vi "Send Packet.vi"(6 "timeout (0ms : no ack)":i32, 8 "error in (no error)":errorcluster, 10 "Packet":refnum<class "ControlPacket.lvclass">, 11 "Session in":refnum<class "Session.lvclass">) -> (0 "error out":errorcluster, 1 "validated":bool, 2 "Response":refnum<class "ControlPacket.lvclass">[](array[class]), 3 "Session out":refnum<class "Session.lvclass">)   [LabVIEW 2013, in "MQTT Server.lvlib" / "Session.lvclass"]
uses:
  Session.lvclass
  Control Packets/ControlPacket/ControlPacket.lvclass
  MQTT_Base/Response -- cluster.ctl
  Session.lvclass/Session.ctl
  MQTT_Base/MQTT_Base.lvclass
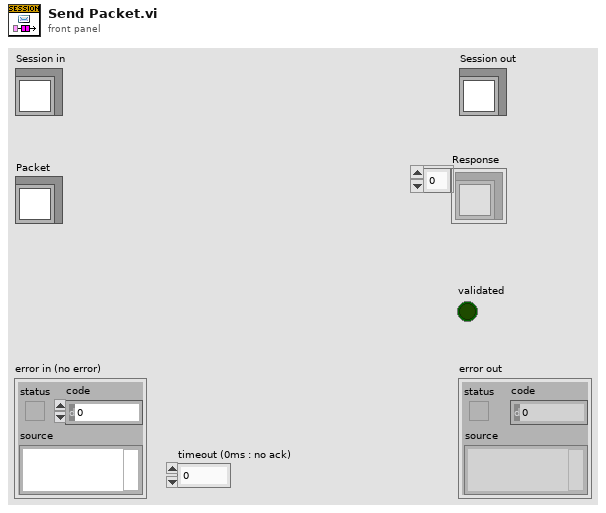
[diagram p1: front panel]
types:
  T1 = typedef "MQTT Server.lvlib/MQTT_Base.lvclass/Response -- cluster.ctl" = cluster{"Packet":refnum<class "ControlPacket.lvclass">, "Protocol Error":errorcluster, "disconnect session":bool, "[ACK]":refnum<notifier>[]}
  T2 = typedef "ControlPacket.lvclass/Control Packet Type -- enum.ctl" = enum16{"Reserved", "CONNECT", "CONNACK", "PUBLISH", "PUBACK", "PUBREC", "PUBREL", "PUBCOMP", "SUBSCRIBE", "SUBACK", "UNSUBSCRIBE", "UNSUBACK", "PINGREQ", "PINGRESP", "DISCONNECT", "Reserved(15)"}
  T3 = typedef "ControlPacket.lvclass/QualityOfService -- enum.ctl" = enum16{"0 (At Most Once)", "1 (At Least Once)", "2 (Exactly Once)"}
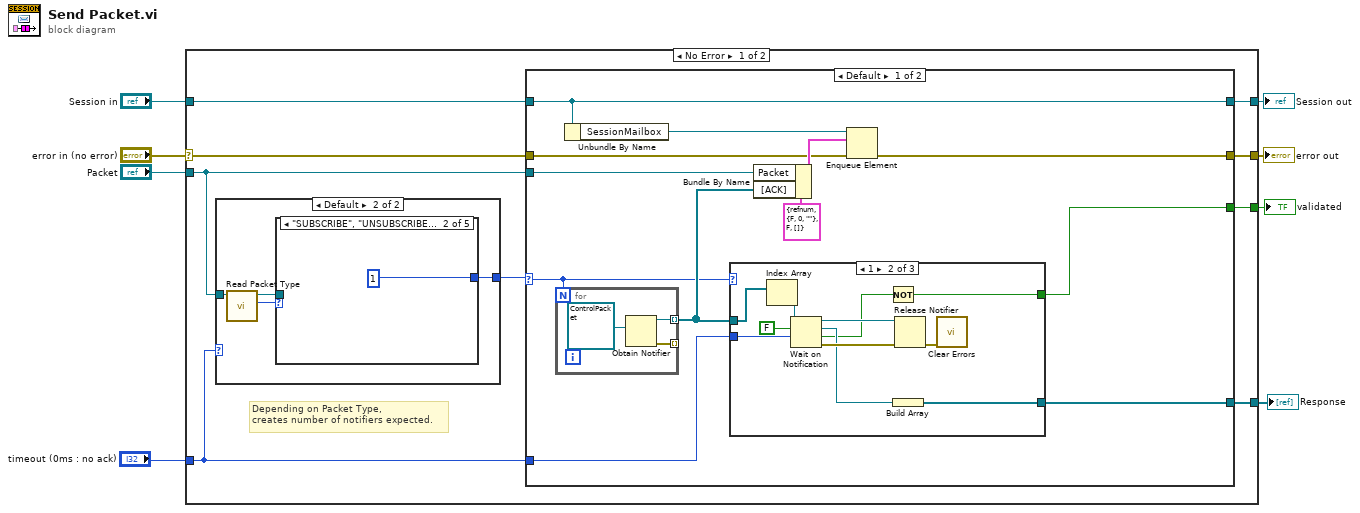
[diagram p0: block diagram]
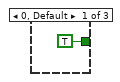
[diagram p2: hidden frame]
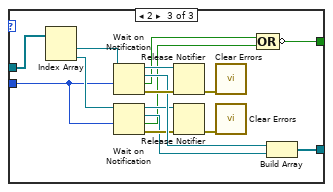
[diagram p3: hidden frame]
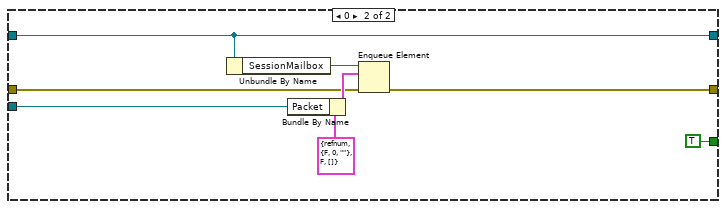
[diagram p4: hidden frame]
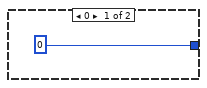
[diagram p5: hidden frame]
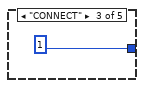
[diagram p7: hidden frame]
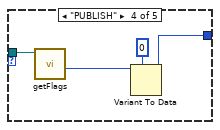
[diagram p8: hidden frame]
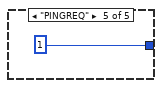
[diagram p9: hidden frame]
diagram:
  n1 = case shown="No Error" "error in (no error)" {
    selector: "error in (no error)" -> [w12 w82]
    tunnel: [w11 w82] -> w7
    tunnel: [w10 w81] -> w5
    tunnel: "Session in" -> [w16 w81]
    tunnel: "Packet" -> [w17 _]
    tunnel: [w13 _] -> w3
    tunnel: "timeout (0ms : no ack)" -> [w15 _]
    tunnel: [w14 _] -> w1
    frame No Error {
      # "Depending on Packet Type, \ncreates number of notifiers expected."
      n2 = case shown="Default" w15 {
        tunnel: w17 -> [_ w73]
        tunnel: [0 w70] -> w9
        frame 0 {
        }
        frame Default {
          n3 = call "Read Packet Type.vi"("ControlPacket in"=w73) -> ("Control Packet Type"=w71:T2, "ControlPacket out"=w72:refnum<class "ControlPacket.lvclass">)  [unwired: 9 in]
          n4 = case shown="\"SUBSCRIBE\", \"UNSUBSCRIBE\"" w71 {
            tunnel: w72 -> [_ _ _ w78 _]
            tunnel: [_ 1 1 w77 1] -> w70
            frame Default {
            }
            frame "SUBSCRIBE", "UNSUBSCRIBE" {
            }
            frame "CONNECT" {
            }
            frame "PUBLISH" {
              n5 = call-dynamic "getFlags.vi"("ControlPacket in"=w78) -> ("QoS"=w76:T3)  [unwired: 7 in, 3 out]
              n6 = Variant To Data(type=0, Variant=w76) -> (data=w77:i32)  [unwired: 1 in, 1 out]
            }
            frame "PINGREQ" {
            }
          }
        }
      }
      n7 = case shown="Default" w9 {
        selector: w9 -> [w20 _]
        tunnel: w17 -> [w29 w68]
        tunnel: w16 -> [w25 w63]
        tunnel: w15 -> [w24 _]
        tunnel: [w21 _] -> w14
        tunnel: [w18 TRUE] -> w13
        tunnel: w12 -> [w19 w62]
        tunnel: [w22 w64] -> w11
        tunnel: [w25 w63] -> w10
        frame Default {
          n8 = for {
            N: w20 -> [_]
            tunnel: [w60] -> _ mode=indexing
            tunnel: [w59] -> w23 mode=indexing
            n9 = Obtain Notifier(notification data type=refnum<class "ControlPacket.lvclass"> refnum ("Ack")) -> (notifier out=w59:refnum<notifier>, error out=w60:errorcluster)  [unwired: 3 in, 1 out]
          }
          n10 = Unbundle By Name(w25) -> ("SessionMailbox"=w28:refnum<queue>)
          n11 = case shown="1" w20 {
            tunnel: w24 -> [_ w41 w45]
            tunnel: w23 -> [_ w36 w54]
            tunnel: [_ w33 w51] -> w21
            tunnel: [TRUE w31 w42] -> w18
            frame 0, Default {
            }
            frame 1 {
              n12 = Index Array(array=w36) -> (element=w35:refnum<notifier>)  [unwired: 1 in]
              n13 = Wait on Notification(notifier=w35, ignore previous (F)=FALSE, timeout in ms (-1)=w41) -> (notifier out=w38:refnum<notifier>, notification=w37:refnum<class "ControlPacket.lvclass">, timed out?=w32:bool, error out=w39:errorcluster)  [unwired: 1 in]
              n14 = Not(x=w32) -> (.not. x?=w31:bool)
              n15 = Build Array(w37) -> (w33:refnum<class "ControlPacket.lvclass">[])
              n16 = Release Notifier(notifier=w38, error in (no error)=w39) -> (error out=w34:errorcluster)  [unwired: 1 in, 2 out]
              n17 = call <vilib>:"Clear Errors.vi"("error in (no error)"=w34) -> ()  [unwired: 6 in, 1 out]
            }
            frame 2 {
              n18 = Index Array(array=w54) -> (element #1=w53:refnum<notifier>, element #2=w47:refnum<notifier>)  [unwired: 2 in]
              n19 = Wait on Notification(notifier=w53, timeout in ms (-1)=w45) -> (notifier out=w56:refnum<notifier>, notification=w55:refnum<class "ControlPacket.lvclass">, timed out?=w44:bool, error out=w57:errorcluster)  [unwired: 2 in]
              n20 = Wait on Notification(notifier=w47, timeout in ms (-1)=w45) -> (notifier out=w46:refnum<notifier>, notification=w48:refnum<class "ControlPacket.lvclass">, timed out?=w43:bool, error out=w49:errorcluster)  [unwired: 2 in]
              n21 = Release Notifier(notifier=w56, error in (no error)=w57) -> (error out=w52:errorcluster)  [unwired: 1 in, 2 out]
              n22 = Release Notifier(notifier=w46, error in (no error)=w49) -> (error out=w50:errorcluster)  [unwired: 1 in, 2 out]
              n23 = call <vilib>:"Clear Errors.vi"("error in (no error)"=w52) -> ()  [unwired: 6 in, 1 out]
              n24 = call <vilib>:"Clear Errors.vi"("error in (no error)"=w50) -> ()  [unwired: 6 in, 1 out]
              n25 = Compound Arithmetic op=OR(w44, w43) -> (invert w42:bool)
              n26 = Build Array(w55, w48) -> (w51:refnum<class "ControlPacket.lvclass">[])
            }
          }
          n27 = Bundle By Name(cluster=T1 {"Packet"=refnum, "Protocol Error"={"status"=FALSE, "code"=0, "source"=""}, "disconnect session"=FALSE, "[ACK]"=[]} ("element"), "Packet"=w29, "[ACK]"=w23) -> (w26:T1)
          n28 = Enqueue Element(queue=w28, element=w26, error in (no error)=w19) -> (error out=w22:errorcluster)  [unwired: 1 in, 2 out]
        }
        frame 0 {
          n29 = Unbundle By Name(w63) -> ("SessionMailbox"=w67:refnum<queue>)
          n30 = Bundle By Name(cluster=T1 {"Packet"=refnum, "Protocol Error"={"status"=FALSE, "code"=0, "source"=""}, "disconnect session"=FALSE, "[ACK]"=[]} ("element"), "Packet"=w68) -> (w65:T1)
          n31 = Enqueue Element(queue=w67, element=w65, error in (no error)=w62) -> (error out=w64:errorcluster)  [unwired: 1 in, 2 out]
        }
      }
    }
    frame Error {
    }
  }
  "error out" <- w7
  "Session out" <- w5
  "validated" <- w3
  "Response" <- w1
